vi "Begin.vi"() -> (0 "error out":errorcluster)   [LabVIEW 2013]
doc: "Called before other user functions, this VI is expected to open initial I/O refnums, load in file data, and do all program initialization. Notice that the <B>error out</B> terminal is simply used for data flow. Wiring it to other structures or subVIs ensures that this VI runs first."
uses:
  <vilib>/Rock Robotics/WPI/DriverStation/WPI_DriverStationRobotMode2.ctl
  Systems/DriverStation/DriverStation.lvclass
  Systems/Shifter/Shifter.lvclass
  Systems/Compressor/Compressor.lvclass
  Systems/GrabberArms/GrabberArms.lvclass
  Systems/GrabberWheels/GrabberWheels.lvclass
  Systems/Catapult/Catapult.lvclass
  Systems/Blocker/Blocker.lvclass
  Systems/DriveMotors/DriveMotors.lvclass
  Robot Global Data.vi
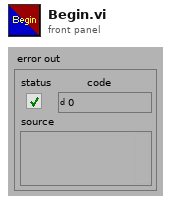
[diagram p1: front panel]
types:
  T1 = typedef "WPI_DriverStationRobotMode2.ctl" = enum16{"Autonomous Disabled", "Autonomous Enabled", "Teleop Disabled", "Teleop Enabled", "Timeout", "Finish", "Test Disabled", "Test Enabled"}
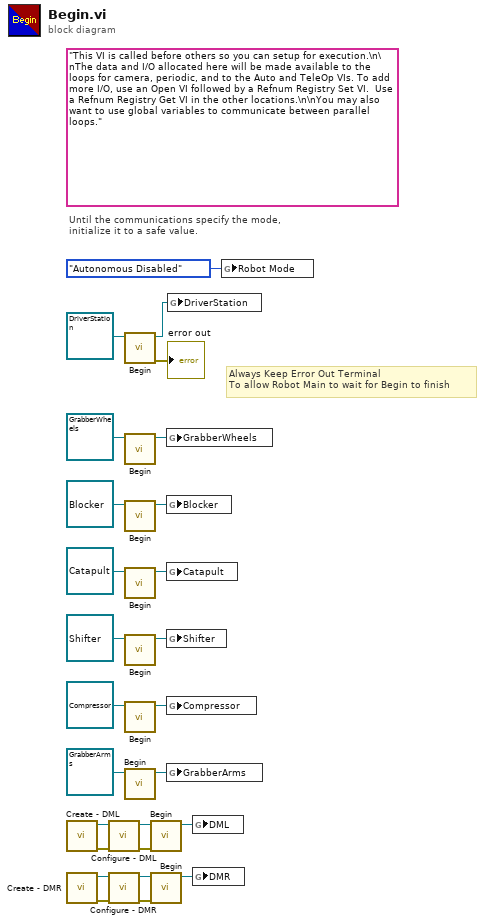
[diagram p0: block diagram]
diagram:
  (unwired) "This VI is called before others so you can setup for execution.\n\nThe data and I/O allocated here will be made available to the loops for camera, periodic, and to the Auto and TeleOp VIs. To add more I/O, use an Open VI followed by a Refnum Registry Set VI.  Use a Refnum Registry Get VI in the other locations.\n\nYou may also want to use global variables to communicate between parallel loops."
  # "Always Keep Error Out Terminal \nTo allow Robot Main to wait for Begin to finish"
  # "Until the communications specify the mode,\ninitialize it to a safe value."
  n1 = call "Create - DML.vi"() -> ("error out"=w8:errorcluster, "DriveMotors out"=w10:refnum<class "DriveMotors.lvclass">)  [unwired: 10 in]
  n2 = call "Create - DMR.vi"() -> ("error out"=w6:errorcluster, "DriveMotors out"=w4:refnum<class "DriveMotors.lvclass">)  [unwired: 10 in]
  n3 = call "Configure - DML.vi"("error in (no error)"=w8, "DriveMotors in"=w10) -> ("error out"=w7:errorcluster, "DriveMotors out"=w9:refnum<class "DriveMotors.lvclass">)  [unwired: 8 in]
  n4 = call "Configure - DMR.vi"("error in (no error)"=w6, "DriveMotors in"=w4) -> ("error out"=w5:errorcluster, "DriveMotors out"=w3:refnum<class "DriveMotors.lvclass">)  [unwired: 8 in]
  n5 = call-dynamic "Begin.vi"("DriverStation in"=refnum<class "DriverStation.lvclass"> refnum ("DriverStation.lvclass")) -> ("error out"=→"error out":errorcluster, "DriverStation out"=w25:refnum<class "DriverStation.lvclass">)  [unwired: 9 in]
  n6 = call-dynamic "Begin.vi"("GrabberWheels in"=refnum<class "GrabberWheels.lvclass"> refnum ("GrabberWheels.lvclass")) -> ("GrabberWheels out"=w15:refnum<class "GrabberWheels.lvclass">)  [unwired: 9 in, 1 out]
  n7 = call-dynamic "Begin.vi"("Blocker in"=refnum<class "Blocker.lvclass"> refnum ("Blocker.lvclass")) -> ("Blocker out"=w1:refnum<class "Blocker.lvclass">)  [unwired: 9 in, 1 out]
  n8 = call-dynamic "Begin.vi"("Catapult in"=refnum<class "Catapult.lvclass"> refnum ("Catapult.lvclass")) -> ("Catapult out"=w13:refnum<class "Catapult.lvclass">)  [unwired: 9 in, 1 out]
  n9 = call-dynamic "Begin.vi"("Shifter in"=refnum<class "Shifter.lvclass"> refnum ("Shifter.lvclass")) -> ("Shifter out"=w21:refnum<class "Shifter.lvclass">)  [unwired: 9 in, 1 out]
  n10 = call-dynamic "Begin.vi"("Compressor in"=refnum<class "Compressor.lvclass"> refnum ("Compressor.lvclass")) -> ("Compressor out"=w19:refnum<class "Compressor.lvclass">)  [unwired: 9 in, 1 out]
  n11 = call-dynamic "Begin.vi"("GrabberArms in"=refnum<class "GrabberArms.lvclass"> refnum ("GrabberArms.lvclass")) -> ("GrabberArms out"=w17:refnum<class "GrabberArms.lvclass">)  [unwired: 9 in, 1 out]
  n12 = call-dynamic "Begin.vi"("error in (no error)"=w7, "DriveMotors in"=w9) -> ("DriveMotors out"=w12:refnum<class "DriveMotors.lvclass">)  [unwired: 8 in, 1 out]
  n13 = call-dynamic "Begin.vi"("error in (no error)"=w5, "DriveMotors in"=w3) -> ("DriveMotors out"=w11:refnum<class "DriveMotors.lvclass">)  [unwired: 8 in, 1 out]
  n14 = global write "Robot Global Data.vi" "GrabberWheels"(w15) -> ()
  n15 = global write "Robot Global Data.vi" "Blocker"(w1) -> ()
  n16 = global write "Robot Global Data.vi" "Catapult"(w13) -> ()
  n17 = global write "Robot Global Data.vi" "Shifter"(w21) -> ()
  n18 = global write "Robot Global Data.vi" "Compressor"(w19) -> ()
  n19 = global write "Robot Global Data.vi" "GrabberArms"(w17) -> ()
  n20 = global write "Robot Global Data.vi" "DriverStation"(w25) -> ()
  n21 = global write "Robot Global Data.vi" "DML"(w12) -> ()
  n22 = global write "Robot Global Data.vi" "DMR"(w11) -> ()
  n23 = global write "Robot Global Data.vi" "Robot Mode"(WPI_DriverStationRobotMode2."Autonomous Disabled" ("Robot Mode")) -> ()
